vi "Main_pro.vi"() -> ()   [LabVIEW 2019]
uses:
  GlobalVar.vi
  <vilib>/addons/control/pid/NI_PID_pid.lvlib
  <vilib>/addons/control/pid/pid.llb/PID (DBL).vi
  <vilib>/myRIO/Common/Instrument Driver Framework/myRIO v1.0/Encoder/typedefs/Encoder Count Direction Enum.ctl
  <vilib>/myRIO/Common/Instrument Driver Framework/myRIO v1.0/Encoder/typedefs/Encoder Signal Mode.ctl
  <vilib>/myRIO/Common/Instrument Driver Framework/myRIO v1.0/Encoder/typedefs/Encoder Channels Enum.ctl
  <vilib>/myRIO/Common/Instrument Driver Framework/Utilities/typedefs/Generic FPGA Reference.ctl
  <vilib>/myRIO/Common/Instrument Driver Framework/Utilities/typedefs/myRIO v1.0 Reference.ctl
  <vilib>/myRIO/Common/Instrument Driver Framework/Utilities/typedefs/Hardware Version Enum.ctl
  <vilib>/myRIO/Common/Instrument Driver Framework/Utilities/typedefs/myRIO Generic Hardware Reference.ctl
  <vilib>/myRIO/Instrument Drivers/Onboard IO/Encoder/typedefs/Encoder Reference.ctl
  <vilib>/myRIO/Instrument Drivers/Onboard IO/Encoder/Encoder.lvlib
  <vilib>/myRIO/Instrument Drivers/Onboard IO/Encoder/vis/Read.vi
  <vilib>/myRIO/Common/Instrument Driver Framework/myRIO v1.0/Encoder/typedefs/Encoder Configuration v1.0.ctl
  <vilib>/userDefined/High Color/nirio_resource_hc.ctl
  <vilib>/myRIO/Common/Instrument Driver Framework/myRIO v1.0/Encoder/vis/myRIO v1.1 Open Encoder.vi
  <vilib>/myRIO/Common/Instrument Driver Framework/myRIO v1.0/Encoder/vis/myRIO v1.0 Configure Encoder.vi
  <vilib>/myRIO/Instrument Drivers/Onboard IO/Encoder/vis/myRIO Encoder Open.xnode
  <vilib>/myRIO/Common/Instrument Driver Framework/Utilities/vis/Is FPGA Ref Available.vi
  <vilib>/myRIO/Express VI/Onboard IO/Encoder/Encoder Express VI.xnode
  <vilib>/myRIO/Common/Instrument Driver Framework/myRIO v1.0/DIO/typedefs/DIO Channels Enum.ctl
  <vilib>/myRIO/Common/Instrument Driver Framework/myRIO v1.0/DIO/typedefs/DIO Channels List.ctl
  <vilib>/myRIO/Instrument Drivers/Onboard IO/DIO/typedefs/DIO Reference.ctl
  <vilib>/myRIO/Instrument Drivers/Onboard IO/DIO/DIO.lvlib
  <vilib>/myRIO/Instrument Drivers/Onboard IO/DIO/vis/Write.vi
  <vilib>/myRIO/Common/Instrument Driver Framework/myRIO v1.0/DIO/vis/myRIO v1.1 Open DIO.vi
  <vilib>/myRIO/Instrument Drivers/Onboard IO/DIO/vis/myRIO DIO Open.xnode
  <vilib>/myRIO/Express VI/Onboard IO/DO/DO Express VI.xnode
  <vilib>/robotics/Steering/Steering Frame/NI_Robotics_Steering Frame.lvclass
panel:
  in  "element 3":dbl
  in  "element 2":dbl
  in  "element":dbl
  out "error out":errorcluster
  out "Pps_M 3":i32
  out "Pps_M 2":i32
  out "Pps_M 1":i32
  in  "output range Theta":cluster{"output high":dbl, "output low":dbl}={"output high"=180.0, "output low"=-180.0} {"output low" format="%.2f"; "output high" format="%.2f"}
  in  "output range Y":cluster{"output high":dbl, "output low":dbl}={"output high"=1500.0, "output low"=-1500.0} {"output low" format="%.2f"; "output high" format="%.2f"}
  in  "output range X":cluster{"output high":dbl, "output low":dbl}={"output high"=1500.0, "output low"=-1500.0} {"output low" format="%.2f"; "output high" format="%.2f"}
  in  "Test_X":bool
  in  "Test_Theta":bool
  in  "Test_Y":bool
  out "Theta":cluster{"Theta set":dbl, "ThetaHead_En":dbl}(graph)
  out "Y":cluster{"Y Set":dbl, "Y_En":dbl}(graph)
  out "X":cluster{"X Set":dbl, "X_En":dbl}(graph)
  in  "Param PID Y":T1={"proportional gain (Kc)"=1.0, "integral time (Ti, min)"=0.0, "derivative time (Td, min)"=0.0} {"derivative time (Td, min)" format="%.5f"; "integral time (Ti, min)" format="%.5f"; "proportional gain (Kc)" format="%.5f"}
  out "PIDY":dbl
  in  "Param PID Theta":T1={"proportional gain (Kc)"=1.0, "integral time (Ti, min)"=0.0, "derivative time (Td, min)"=0.0} {"derivative time (Td, min)" format="%.5f"; "integral time (Ti, min)" format="%.5f"; "proportional gain (Kc)" format="%.5f"}
  out "PIDTheta":dbl
  out "PIDX":dbl
  in  "Param PID X":T1={"proportional gain (Kc)"=1.0, "integral time (Ti, min)"=0.0, "derivative time (Td, min)"=0.0} {"derivative time (Td, min)" format="%.5f"; "integral time (Ti, min)" format="%.5f"; "proportional gain (Kc)" format="%.5f"}
  out "millisecond timer value":u32
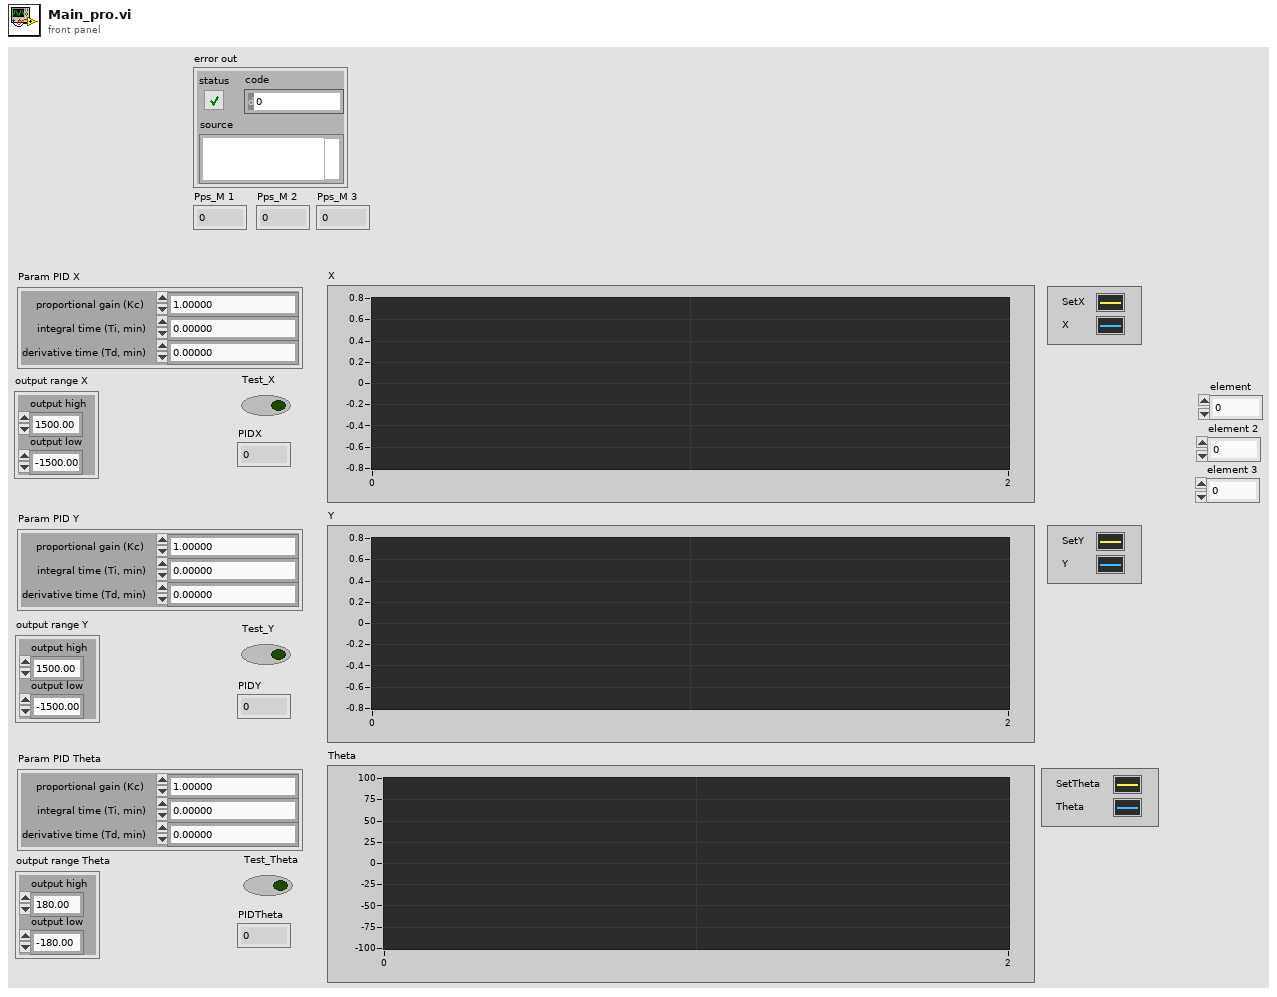
[diagram p1: front panel]
types:
  T1 = cluster{"proportional gain (Kc)":dbl, "integral time (Ti, min)":dbl, "derivative time (Td, min)":dbl}
  T2 = typedef "DIO.lvlib/DIO Reference.ctl" = cluster{"myRIO Reference":T3, "DIO Channels List":T7}
  T3 = typedef "myRIO Generic Hardware Reference.ctl" = cluster{"myRIO Model":T4, "myRIO Hardware Reference":T5}
  T4 = typedef "Hardware Version Enum.ctl" = enum16{"Unknown", "myRIO-1900", "myRIO-1950", "roboRIO", "NI ELVIS RIO CM", "ELVIS III"}
  T5 = typedef "myRIO v1.0 Reference.ctl" = cluster{"Generic FPGA Reference":T6, "Allow multiple opens":bool}
  T6 = typedef "Generic FPGA Reference.ctl" = refnum<k20>
  T7 = typedef "DIO Channels List.ctl" = T8[]
  T8 = typedef "DIO Channels Enum.ctl" = enum16{"Not Connected", "C/DIO0", "C/DIO1", "C/DIO2", "C/DIO3", "C/DIO4", "C/DIO5", "C/DIO6", "C/DIO7", "A/DIO0", "A/DIO1", "A/DIO2", "A/DIO3", "A/DIO4", "A/DIO5", "A/DIO6", "A/DIO7", "A/DIO8", "A/DIO9", "A/DIO10", "A/DIO11", "A/DIO12", "A/DIO13", "A/DIO14", "A/DIO15", "A/DIO16", "A/DIO17", "A/DIO18", "A/DIO19", "B/DIO0", "B/DIO1", "B/DIO2", "B/DIO3", "B/DIO4", "B/DIO5", "B/DIO6", "B/DIO7", "B/DIO8", "B/DIO9", "B/DIO10", "B/DIO11", "B/DIO12", "B/DIO13", "B/DIO14", "B/DIO15", "B/DIO16", "B/DIO17", "B/DIO18", "B/DIO19", "LED0", "LED1", "LED2", "LED3", "Button0", "DIO/DIO0", "DIO/DIO1", "DIO/DIO2", "DIO/DIO3", "DIO/DIO4", "DIO/DIO5", "DIO/DIO6", "DIO/DIO7", "DIO/DIO8", "DIO/DIO9", "SPI/CS0", "SPI/CS1", "SPI/CS2", "SPI/CS3", "LED RADIO (Green)", "LED RADIO (Red)", "LED COMM (Green)", "LED COMM (Red)", "LED MODE (Green)", "LED MODE (Red)"}
  T9 = typedef "nirio_resource_hc.ctl" = tag
  T10 = typedef "Encoder.lvlib/Encoder Reference.ctl" = cluster{"myRIO Reference":T3, "Encoder Channels Enum":T11}
  T11 = typedef "Encoder Channels Enum.ctl" = enum16{"Not Connected", "C/ENC0", "C/ENC1", "A/ENC", "A/ENC0", "A/ENC1", "A/ENC2", "A/ENC3", "A/ENC4", "A/ENC5", "A/ENC6", "A/ENC7", "A/ENC8", "A/ENC9", "B/ENC", "B/ENC0", "B/ENC1", "B/ENC2", "B/ENC3", "B/ENC4", "B/ENC5", "B/ENC6", "B/ENC7", "B/ENC8", "B/ENC9", "DIO/ENC0", "DIO/ENC1", "DIO/ENC2", "DIO/ENC3", "DIO/ENC4"}
  T12 = typedef "Encoder Signal Mode.ctl" = enum16{"Quadrature phase signal", "Step and direction signal"}
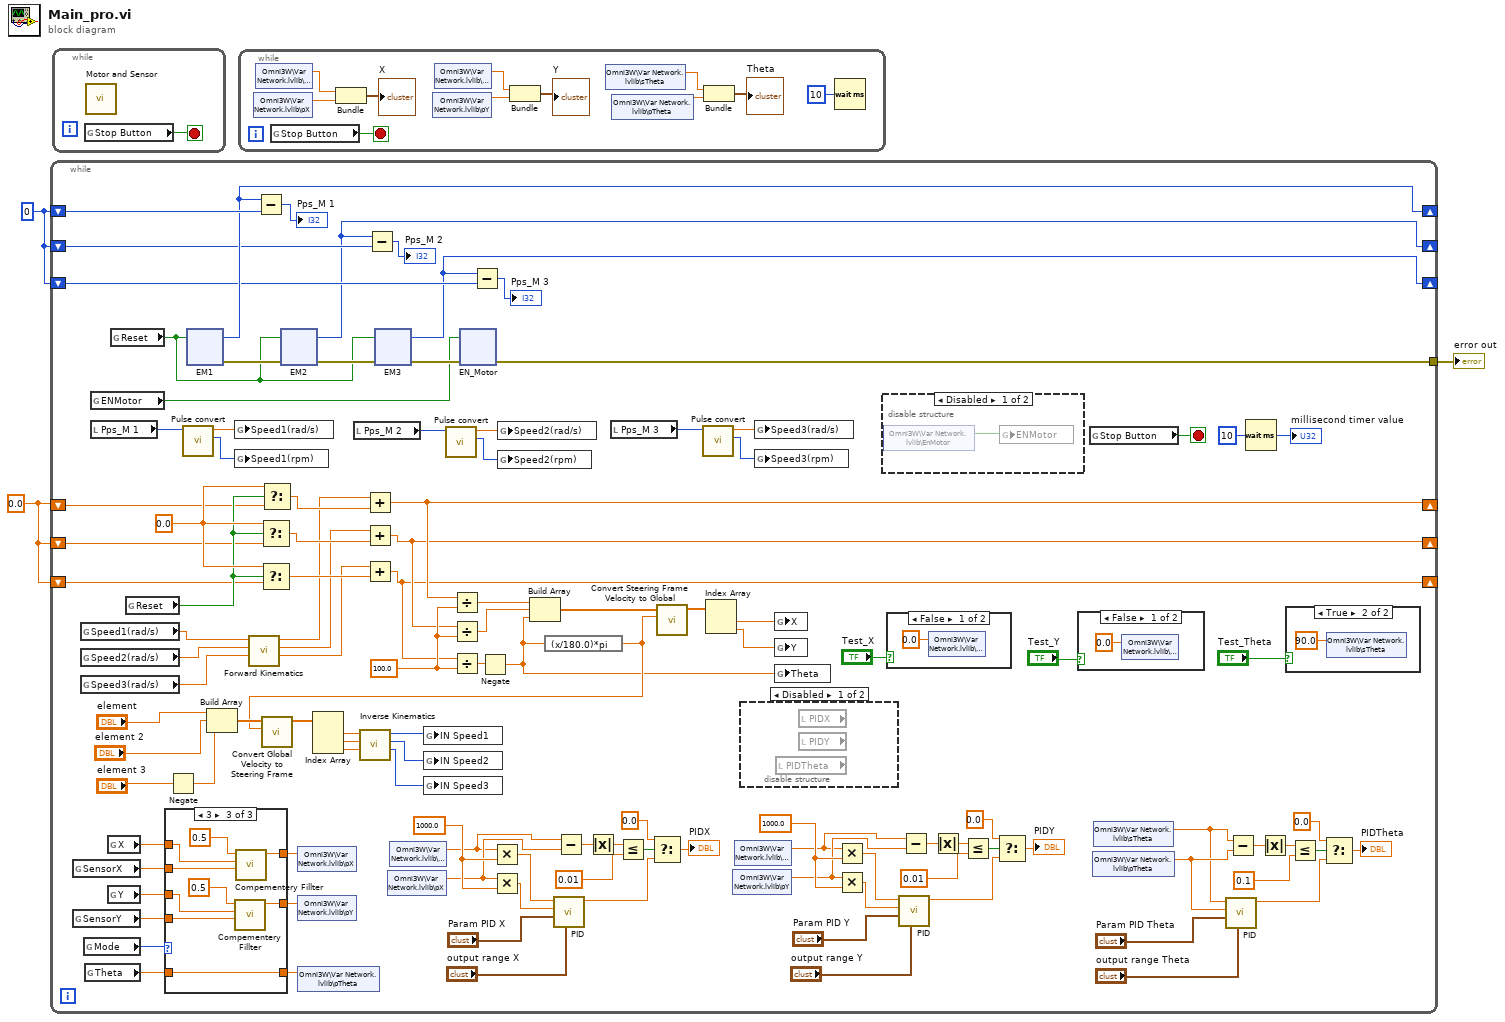
[diagram p0: block diagram]
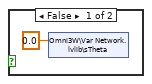
[diagram p4: hidden frame]
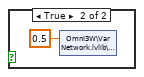
[diagram p5: hidden frame]
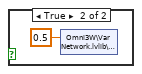
[diagram p6: hidden frame]
diagram:
  w2 = 0
  w3 = 0.0
  n1 = while {
    shift-right: [w104] -> _
    shift-left: w3 -> [w117]
    shift-right: [w103] -> _
    shift-left: w3 -> [w116]
    shift-right: [w102] -> _
    shift-left: w3 -> [w115]
    shift-right: [w32] -> _
    shift-left: w2 -> [w33]
    shift-right: [w28] -> _
    shift-left: w2 -> [w31]
    shift-right: [w27] -> _
    shift-left: w2 -> [w30]
    tunnel: [w29] -> w1
    stop <- w120 stop-if-true
    w69 = 1000.0 ("y")
    w74 = 1000.0 ("y")
    w105 = 100.0 ("y")
    w119 = 0.0 ("t")
    n2 = global read "GlobalVar.vi" "SensorX"() -> (w96:dbl)
    n3 = global read "GlobalVar.vi" "SensorY"() -> (w94:dbl)
    n4 = global read "GlobalVar.vi" "Speed1(rad/s)"() -> (w114:dbl)
    n5 = global read "GlobalVar.vi" "Speed2(rad/s)"() -> (w113:dbl)
    n6 = global read "GlobalVar.vi" "Speed3(rad/s)"() -> (w112:dbl)
    n7 = global read "GlobalVar.vi" "Mode"() -> (w99:i8)
    n8 = global read "GlobalVar.vi" "Theta"() -> (w98:dbl)
    n9 = global read "GlobalVar.vi" "ENMotor"() -> (w46:bool)
    n10 = local read "Pps_M 1"() -> (w45:i32)
    n11 = global read "GlobalVar.vi" "X"() -> (w97:dbl)
    n12 = global read "GlobalVar.vi" "Y"() -> (w95:dbl)
    n13 = global read "GlobalVar.vi" "Reset"() -> (w47:bool)
    n14 = global read "GlobalVar.vi" "Reset"() -> (w118:bool)
    n15 = case shown="3" w99 {
      tunnel: w98 -> [w301 w304 w307]
      tunnel: w97 -> [w303 _ w313]
      tunnel: w96 -> [_ w306 w312]
      tunnel: w95 -> [w302 _ w311]
      tunnel: w94 -> [_ w305 w310]
      tunnel: [w303 w306 w309] -> w93
      tunnel: [w302 w305 w308] -> w92
      tunnel: [w301 w304 w307] -> w91
      frame 1, Default {
      }
      frame 2 {
      }
      frame 3 {
        n16 = call "Compementery Fillter.vi"("data2"=w310, "data1"=w311, "a"=0.5) -> ("DataOut"=w308:dbl)  [unwired: 8 in]
        n17 = call "Compementery Fillter.vi"("data2"=w312, "data1"=w313, "a"=0.5) -> ("DataOut"=w309:dbl)  [unwired: 8 in]
      }
    }
    n18 = Negate(x="element 3") -> (-x=w8:dbl)
    n19 = call "Pulse convert.vi"("PulseIN"=w45) -> ("Speed(rpm)"=w43:i16, "Speed(rad/s)"=w44:dbl)  [unwired: 9 in]
    n20 = xnode "EM1"("Reset Counter"=w47) -> ("error out"=w50:errorcluster, "Counter Value"=w32:i32)  [unwired: 1 in, 2 out]
    n21 = Build Array("element", "element 2", w8) -> (w15:dbl[])
    n22 = global write "GlobalVar.vi" "Speed1(rad/s)"(w44) -> ()
    n23 = global write "GlobalVar.vi" "Speed1(rpm)"(w43) -> ()
    n24 = call "Forward Kinematics.vi"("Phi3(rad/s)"=w112, "Phi2(rad/s)"=w113, "Phi1(rad/s)"=w114) -> ("Theta(deg/s)"=w106:dbl, "Y(m/s)"=w107:dbl, "X(m/s)"=w108:dbl)  [unwired: 6 in]
    n25 = Subtract(x=w32, y=w33) -> (x-y=→"Pps_M 1":i32)
    n26 = Select(t=w119, s=w118, f=w116) -> (s? t:f=w110:dbl)
    n27 = Select(t=w119, s=w118, f=w115) -> (s? t:f=w109:dbl)
    n28 = Select(t=w119, s=w118, f=w117) -> (s? t:f=w111:dbl)
    n29 = xnode "EM2"("error in (no error)"=w50, "Reset Counter"=w47) -> ("error out"=w49:errorcluster, "Counter Value"=w28:i32)  [unwired: 2 out]
    n30 = shared-variable "Omni3W\\Var Network.lvlib\\pX"(w93) -> ()  [unwired: 1 in, 1 out]
    n31 = shared-variable "Omni3W\\Var Network.lvlib\\pY"(w92) -> ()  [unwired: 1 in, 1 out]
    n32 = shared-variable "Omni3W\\Var Network.lvlib\\pTheta"(w91) -> ()  [unwired: 1 in, 1 out]
    n33 = local read "Pps_M 2"() -> (w40:i32)
    n34 = Add(x=w108, y=w111) -> (x+y=w104:dbl)
    n35 = Add(x=w107, y=w110) -> (x+y=w103:dbl)
    n36 = Add(x=w106, y=w109) -> (x+y=w102:dbl)
    n37 = Subtract(x=w28, y=w31) -> (x-y=→"Pps_M 2":i32)
    n38 = xnode "EM3"("error in (no error)"=w49, "Reset Counter"=w47) -> ("error out"=w48:errorcluster, "Counter Value"=w27:i32)  [unwired: 2 out]
    n39 = shared-variable "Omni3W\\Var Network.lvlib\\pX"() -> (w57:dbl)  [unwired: 1 in, 1 out]
    n40 = shared-variable "Omni3W\\Var Network.lvlib\\sX"() -> (w56:dbl)  [unwired: 1 in, 1 out]
    n41 = call "Pulse convert.vi"("PulseIN"=w40) -> ("Speed(rpm)"=w42:i16, "Speed(rad/s)"=w41:dbl)  [unwired: 9 in]
    n42 = Divide(x=w104, y=w105) -> (x/y=w20:dbl)
    n43 = Divide(x=w103, y=w105) -> (x/y=w19:dbl)
    n44 = Divide(x=w102, y=w105) -> (x/y=w5:dbl)
    n45 = xnode "EN_Motor"("error in (no error)"=w48, "EN_Motor (A/DIO4 (Pin 19))"=w46) -> ("error out"=w29:errorcluster)
    n46 = Subtract(x=w27, y=w30) -> (x-y=→"Pps_M 3":i32)
    n47 = Negate(x=w5) -> (-x=w4:dbl)
    n48 = Multiply(x=w56, y=w74) -> (x*y=w73:dbl)
    n49 = Multiply(x=w57, y=w74) -> (x*y=w72:dbl)
    n50 = global write "GlobalVar.vi" "Speed2(rad/s)"(w41) -> ()
    n51 = global write "GlobalVar.vi" "Speed2(rpm)"(w42) -> ()
    n52 = Build Array(w20, w19, w4) -> (w18:dbl[])
    n53 = expression code="(x/180.0)*pi" ("degrees to radians")(w4) -> (w6:dbl)
    n54 = call <vilib>:"Convert Global Velocity to Steering Frame.vi"("steering frame angle (rad)"=w6, "global velocity"=w15) -> ("steering frame velocity"=w14:dbl[])  [unwired: 9 in]
    n55 = Index Array(array=w14) -> (element #1=w13:dbl, element #2=w12:dbl, element #3=w11:dbl)  [unwired: 3 in]
    n56 = call "Inverse Kinematics.vi"("Theta Set"=w11, "Y Set"=w12, "X Set"=w13) -> ("Out Motor 3"=w24:i16, "Out Motor 2"=w25:i16, "Out Motor 1"=w26:i16)  [unwired: 6 in]
    n57 = global write "GlobalVar.vi" "IN Speed1"(w26) -> ()
    n58 = global write "GlobalVar.vi" "IN Speed2"(w25) -> ()
    n59 = global write "GlobalVar.vi" "IN Speed3"(w24) -> ()
    n60 = call-poly <vilib>:"PID.vi"("output range"="output range X", "PID gains"="Param PID X", "process variable"=w72, "setpoint"=w73) -> ("output"=w84:dbl)  [unwired: 6 in, 1 out]
    n61 = Subtract(x=w56, y=w57) -> (x-y=w86:dbl)
    n62 = Absolute Value(x=w86) -> (abs(x)=w87:dbl)
    n63 = local read "Pps_M 3"() -> (w39:i32)
    n64 = Less Or Equal?(x=w87, y=0.01) -> (x <= y?=w89:bool)
    n65 = Select(t=0.0, s=w89, f=w84) -> (s? t:f=→"PIDX":dbl)
    n66 = call <vilib>:"Convert Steering Frame Velocity to Global.vi"("steering frame angle (rad)"=w6, "steering frame velocity"=w18) -> ("global velocity"=w21:dbl[])  [unwired: 9 in]
    n67 = call "Pulse convert.vi"("PulseIN"=w39) -> ("Speed(rpm)"=w37:i16, "Speed(rad/s)"=w38:dbl)  [unwired: 9 in]
    n68 = Index Array(array=w21) -> (element #1=w17:dbl, element #2=w16:dbl)  [unwired: 2 in]
    n69 = shared-variable "Omni3W\\Var Network.lvlib\\pY"() -> (w55:dbl)  [unwired: 1 in, 1 out]
    n70 = shared-variable "Omni3W\\Var Network.lvlib\\sY"() -> (w54:dbl)  [unwired: 1 in, 1 out]
    n71 = disable-structure shown="Disabled" {
      frame Disabled {
        n72 = local read "PIDTheta"() -> ()  [unwired: 1 out]
        n73 = local read "PIDX"() -> ()  [unwired: 1 out]
        n74 = local read "PIDY"() -> ()  [unwired: 1 out]
      }
      frame Enabled {
      }
    }
    n75 = global write "GlobalVar.vi" "Speed3(rad/s)"(w38) -> ()
    n76 = global write "GlobalVar.vi" "Speed3(rpm)"(w37) -> ()
    n77 = global write "GlobalVar.vi" "X"(w17) -> ()
    n78 = global write "GlobalVar.vi" "Y"(w16) -> ()
    n79 = global write "GlobalVar.vi" "Theta"(w4) -> ()
    n80 = Multiply(x=w54, y=w69) -> (x*y=w70:dbl)
    n81 = Multiply(x=w55, y=w69) -> (x*y=w71:dbl)
    n82 = disable-structure shown="Disabled" {
      frame Disabled {
        n83 = shared-variable "Omni3W\\Var Network.lvlib\\EnMotor"() -> (w121:bool)  [unwired: 1 in, 1 out]
        n84 = global write "GlobalVar.vi" "ENMotor"(w121) -> ()
      }
      frame Enabled {
      }
    }
    n85 = case shown="False" "Test_X" {
      frame False {
        n86 = shared-variable "Omni3W\\Var Network.lvlib\\sX"(0.0 ("sX")) -> ()  [unwired: 1 in, 1 out]
      }
      frame True {
        n87 = shared-variable "Omni3W\\Var Network.lvlib\\sX"(0.5 ("sX")) -> ()  [unwired: 1 in, 1 out]
      }
    }
    n88 = call-poly <vilib>:"PID.vi"("output range"="output range Y", "PID gains"="Param PID Y", "process variable"=w71, "setpoint"=w70) -> ("output"=w67:dbl)  [unwired: 6 in, 1 out]
    n89 = Subtract(x=w54, y=w55) -> (x-y=w65:dbl)
    n90 = Absolute Value(x=w65) -> (abs(x)=w64:dbl)
    n91 = Less Or Equal?(x=w64, y=0.01) -> (x <= y?=w62:bool)
    n92 = Select(t=0.0, s=w62, f=w67) -> (s? t:f=→"PIDY":dbl)
    n93 = case shown="False" "Test_Y" {
      frame False {
        n94 = shared-variable "Omni3W\\Var Network.lvlib\\sY"(0.0 ("sY")) -> ()  [unwired: 1 in, 1 out]
      }
      frame True {
        n95 = shared-variable "Omni3W\\Var Network.lvlib\\sY"(0.5 ("sY")) -> ()  [unwired: 1 in, 1 out]
      }
    }
    n96 = global read "GlobalVar.vi" "Stop Button"() -> (w120:bool)
    n97 = shared-variable "Omni3W\\Var Network.lvlib\\pTheta"() -> (w81:dbl)  [unwired: 1 in, 1 out]
    n98 = shared-variable "Omni3W\\Var Network.lvlib\\sTheta"() -> (w80:dbl)  [unwired: 1 in, 1 out]
    n99 = call-poly <vilib>:"PID.vi"("output range"="output range Theta", "PID gains"="Param PID Theta", "process variable"=w81, "setpoint"=w80) -> ("output"=w22:dbl)  [unwired: 6 in, 1 out]
    n100 = Subtract(x=w80, y=w81) -> (x-y=w79:dbl)
    n101 = Wait (ms)(milliseconds to wait=u32 10) -> (millisecond timer value=→"millisecond timer value":u32)
    n102 = Absolute Value(x=w79) -> (abs(x)=w78:dbl)
    n103 = case shown="True" "Test_Theta" {
      frame False {
        n104 = shared-variable "Omni3W\\Var Network.lvlib\\sTheta"(0.0 ("sTheta")) -> ()  [unwired: 1 in, 1 out]
      }
      frame True {
        n105 = shared-variable "Omni3W\\Var Network.lvlib\\sTheta"(90.0 ("sTheta")) -> ()  [unwired: 1 in, 1 out]
      }
    }
    n106 = Less Or Equal?(x=w78, y=0.1) -> (x <= y?=w76:bool)
    n107 = Select(t=0.0, s=w76, f=w22) -> (s? t:f=→"PIDTheta":dbl)
  }
  "error out" <- w1
  n108 = while {
    stop <- w316 stop-if-true
    n109 = global read "GlobalVar.vi" "Stop Button"() -> (w316:bool)
    n110 = call "Motor and Sensor.vi"() -> ()  [unwired: 12 in]
  }
  n111 = while {
    stop <- w327 stop-if-true
    n112 = shared-variable "Omni3W\\Var Network.lvlib\\pX"() -> (w324:dbl)  [unwired: 1 in, 1 out]
    n113 = shared-variable "Omni3W\\Var Network.lvlib\\sX"() -> (w325:dbl)  [unwired: 1 in, 1 out]
    n114 = global read "GlobalVar.vi" "Stop Button"() -> (w327:bool)
    n115 = Bundle("Double"=w325, "Double"=w324) -> (→"X":cluster{"Double":dbl, "Double":dbl})  [unwired: 1 in]
    n116 = shared-variable "Omni3W\\Var Network.lvlib\\pY"() -> (w321:dbl)  [unwired: 1 in, 1 out]
    n117 = shared-variable "Omni3W\\Var Network.lvlib\\sY"() -> (w322:dbl)  [unwired: 1 in, 1 out]
    n118 = Bundle("Double"=w322, "Double"=w321) -> (→"Y":cluster{"Double":dbl, "Double":dbl})  [unwired: 1 in]
    n119 = shared-variable "Omni3W\\Var Network.lvlib\\sTheta"() -> (w318:dbl)  [unwired: 1 in, 1 out]
    n120 = shared-variable "Omni3W\\Var Network.lvlib\\pTheta"() -> (w319:dbl)  [unwired: 1 in, 1 out]
    n121 = Bundle("Double"=w318, "Double"=w319) -> (→"Theta":cluster{"Double":dbl, "Double":dbl})  [unwired: 1 in]
    n122 = Wait (ms)(milliseconds to wait=u32 10) -> ()  [unwired: 1 out]
  }
